vi "SYST_SEC_LEV.vi"(0 "VISA IN":refnum<visa-resource-name>, 5 "error in":errorcluster, 7 "Level":string(combo)="None") -> (14 "VISA Out":refnum<visa-resource-name>, 19 "error out":errorcluster)   [LabVIEW 2018, in "PNA-X.lvlib"]
doc: "SYSTem:SECurity[:LEVel] <char> \n(Read-Write) Sets and returns the display of frequency information on the PNA screen and printouts. \nLearn more about security level. \nParameters \n<char> Choose from: \nNone - ALL frequency information is displayed \nLow - NO frequency information is displayed. Frequency information can be \nredisplayed using the Security Setting dialog box or this command.. \nHigh - NO frequency information is displayed. Frequency information can be \nredisplayed ONLY by performing a Preset or recalling an instrument state with \nNone or Low security settings, or using this command. \n1879\n\nExamples SYST:SEC LOW \nsystem:security:level high \nQuery Syntax SYSTem:SECurity[:LEVel]? \nReturn Type Character \nDefault None"
uses:
  PNA-X.lvlib
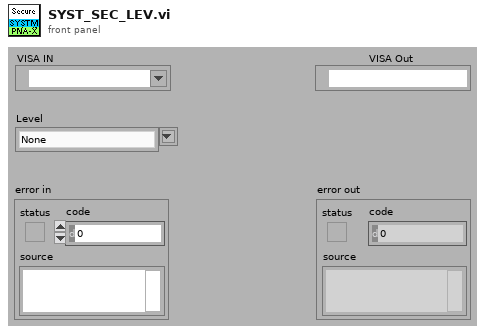
[diagram p1: front panel]
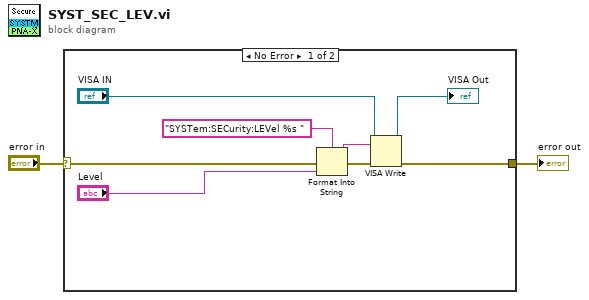
[diagram p0: block diagram]
diagram:
  n1 = case shown="No Error" "error in" {
    selector: "error in" -> [w10 w11]
    tunnel: [w5 w11] -> w1
    frame No Error {
      n2 = Format Into String(format string="SYSTem:SECurity:LEVel %s " ("Cmdline"), error in=w10, "Level") -> (resulting string=w8:string, error out=w9:errorcluster)  [unwired: 1 in]
      n3 = VISA Write(VISA resource name="VISA IN", write buffer=w8, error in (no error)=w9) -> (VISA resource name out=→"VISA Out":refnum<visa-resource-name>, error out=w5:errorcluster)  [unwired: 1 out]
    }
    frame Error {
    }
  }
  "error out" <- w1
